vi "Write New Message Event.vi"(8 "error in (no error)":errorcluster, 10 "New Message Event":refnum<user-event>, 11 "Pub Sub Event Channel in":refnum<class "Pub Sub Event Channel.lvclass">) -> (0 "error out":errorcluster, 3 "Pub Sub Event Channel out":refnum<class "Pub Sub Event Channel.lvclass">)   [LabVIEW 2020, in "Actor Pub Sub Channels.lvlib" / "Pub Sub Event Channel.lvclass"]
uses:
  Pub Sub Event Channel.lvclass
  <vilib>/ActorFramework/Message/Message.lvclass
  Pub Sub Event Channel.lvclass/Pub Sub Event Channel.ctl
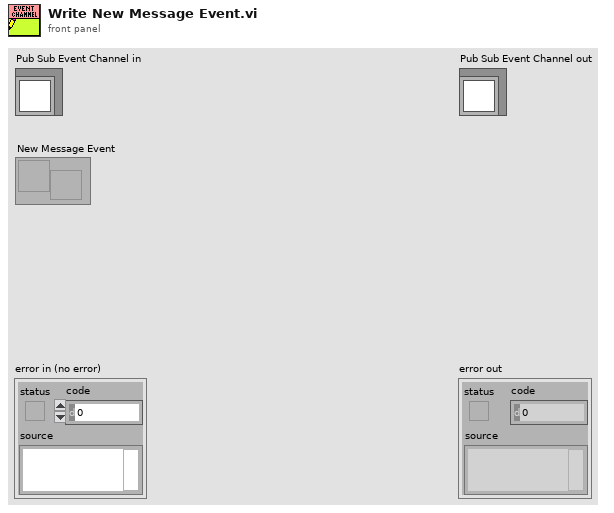
[diagram p1: front panel]
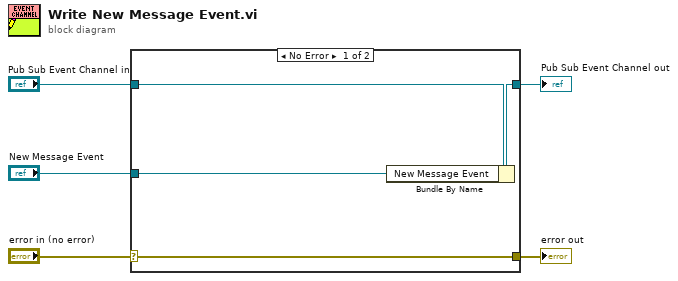
[diagram p0: block diagram]
diagram:
  n1 = case shown="No Error" "error in (no error)" {
    selector: "error in (no error)" -> [w9 w10]
    tunnel: [w9 w10] -> w4
    tunnel: [w7 w11] -> w2
    tunnel: "Pub Sub Event Channel in" -> [w8 w11]
    tunnel: "New Message Event" -> [w6 _]
    frame No Error {
      n2 = Bundle By Name(cluster=w8, "New Message Event"=w6) -> (w7:refnum<class "Pub Sub Event Channel.lvclass">)
    }
    frame Error {
    }
  }
  "error out" <- w4
  "Pub Sub Event Channel out" <- w2
